vi "Get SysDef Path.vi"(11 "Scalar Channels Testing in":refnum<class "Scalar Channels Testing.lvclass">) -> (2 "SysDef Path":path, 3 "Scalar Channels Testing out":refnum<class "Scalar Channels Testing.lvclass">)   [LabVIEW 2019, in "Scalar Channels Testing.lvclass"]
uses:
  Scalar Channels Testing.lvclass
  Scalar Channels Testing.lvclass/Scalar Channels Testing.ctl
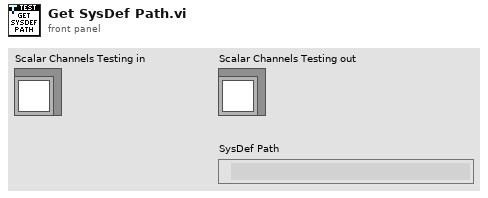
[diagram p1: front panel]
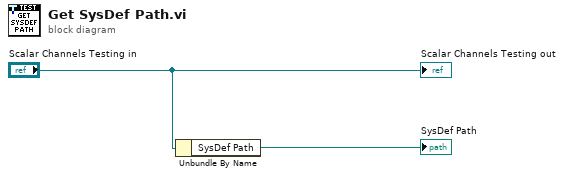
[diagram p0: block diagram]
diagram:
  n1 = Unbundle By Name("Scalar Channels Testing in") -> ("SysDef Path"=→"SysDef Path":path)
  "Scalar Channels Testing out" <- "Scalar Channels Testing in"
